vi "Send onTool.vi"(6 "Tool Data":T1, 8 "error in (no error)":errorcluster, 9 "response":string, 10 "request":string, 11 "id":i32) -> (0 "error out":errorcluster)   [LabVIEW 2025, in "MCP Server.lvlib"]
uses:
  Tool Data.ctl
  Input Parameter.ctl
  Output Parameter.ctl
  onTool.ctl
  MCP Server.lvlib
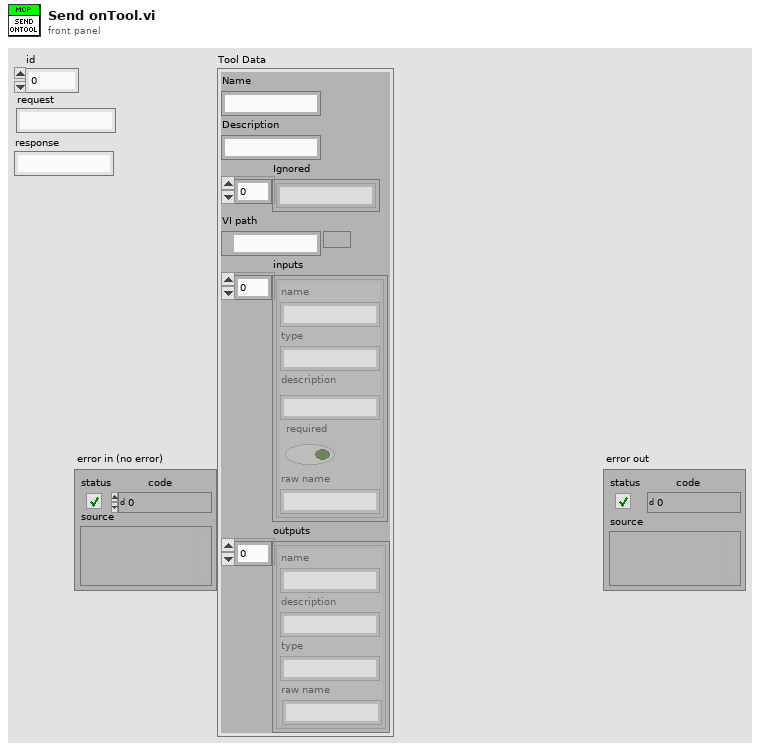
[diagram p1: front panel]
types:
  T1 = typedef "MCP Server.lvlib/Tool Data.ctl" = cluster{"Name":string, "Description":string, "Ignored":string[], "VI path":path, "inputs":T2[], "outputs":T3[]}
  T2 = typedef "MCP Server.lvlib/Input Parameter.ctl" = cluster{"name":string, "type":string, "description":string, "required":bool, "raw name":string}
  T3 = typedef "MCP Server.lvlib/Output Parameter.ctl" = cluster{"name":string, "description":string, "type":string, "raw name":string}
  T4 = typedef "MCP Server.lvlib/onTool.ctl" = cluster{"Tool Data":T1, "request":string, "response":string}
  T5 = typedef "MCP Server.lvlib/Server Data.ctl" = cluster{"Name":string, "Description":string, "Tools":T1[], "Parameters":string[][], "Logging Info":T6, "User Events":T7}
  T6 = typedef "MCP Server.lvlib/Logging.ctl" = cluster{"Log":string[], "Max Length":i32}
  T7 = typedef "MCP Server.lvlib/User Events.ctl" = cluster{"onError":refnum<user-event>, "onLog":refnum<user-event>, "onConnect":refnum<user-event>, "onToolsList":refnum<user-event>, "onToolsCall":refnum<user-event>, "onNotification":refnum<user-event>, "onTool":refnum<user-event>, "onRpc":refnum<user-event>}
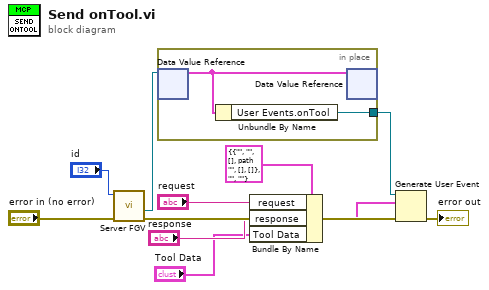
[diagram p0: block diagram]
diagram:
  n1 = call "Server FGV.vi"("error in"="error in (no error)", "id"="id") -> ("error in 2"=w10:errorcluster, "server reference"=w7:refnum<data-value>)  [unwired: 5 in, 3 out]
  n2 = in-place {
    in-place-border: [w12] -> w6
    n3 = in-place-dvr #1(w7) -> (w13:T5)  [unwired: 1 out]
    n4 = Unbundle By Name(w13) -> ("User Events.onTool"=w12:refnum<user-event>)
    n5 = in-place-dvr #1(w13) -> ()  [unwired: 2 out]
  }
  n6 = Bundle By Name(cluster=T4 {"Tool Data"={"Name"="", "Description"="", "Ignored"=[], "VI path"=path "", "inputs"=[], "outputs"=[]}, "request"="", "response"=""} ("event data"), "request"="request", "response"="response", "Tool Data"="Tool Data") -> (w4:T4)
  n7 = Generate User Event(user event=w6, event data cluster=w4, error in=w10) -> (error out=→"error out":errorcluster)  [unwired: 1 in, 1 out]
